vi "Apply TSC Pop Up.vi"(8 "error in":errorcluster, 9 "Material.Details in":T1={"Font Name"="Segoe UI", "Button.Font Size"=30, "Message.Font Size"=30, "Message.Justification"=enum."Center", "Picture Background"=16777216}, 10 "Theme":u16(ring)=3 items=["Light Theme", "Light Medium Contrast", "Light High Contrast", "Dark Theme", "Dark Medium Contrast", "Dark High Constrast"], 11 "Material Theme in":refnum<class "Material Theme.lvclass">) -> (0 "error out":errorcluster, 1 "Material.Details out":T1={"Font Name"="Segoe UI", "Button.Font Size"=30, "Message.Font Size"=30, "Message.Justification"=enum."Center", "Picture Background"=16777216}, 2 "Material.Scheme out":T2)   [LabVIEW 2021, in "TSC Material Theme.lvlib" / "Material Theme.lvclass"]
doc: "Apply a loaded theme to the TSC Pop Up Library.\n\nhttps://github.com/danielcoons/tsc-pop-up\n\n<b>Code Developed By:</b> +\nDaniel Coons +\nTechnology Service Corporation +\nwww.tsc.com/atcs"
uses:
  Material Theme.lvclass
  Material-Scheme/Material-Scheme.lvclass/Material-Scheme.ctl
  Material Theme.lvclass/Material Theme.ctl
  Material-Scheme/Material-Scheme.lvclass
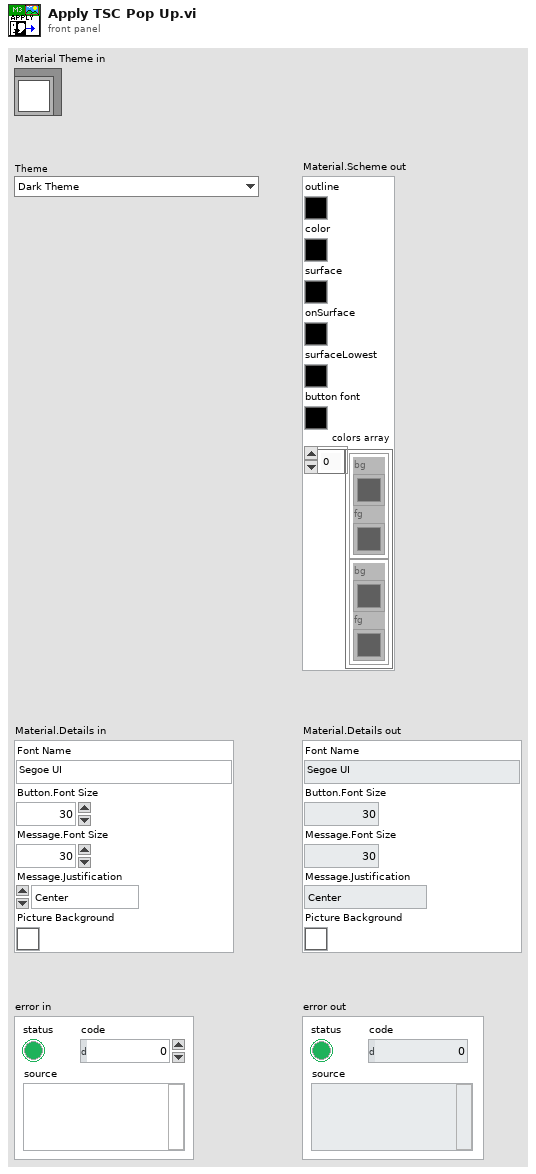
[diagram p1: front panel]
types:
  T1 = cluster{"Font Name":string, "Button.Font Size":u32, "Message.Font Size":u32, "Message.Justification":enum16{"Left", "Center", "Right"}, "Picture Background":u32}
  T2 = cluster{"outline":u32, "color":u32, "surface":u32, "onSurface":u32, "surfaceLowest":u32, "button font":u32, "colors array":cluster{"bg":u32, "fg":u32}[]}
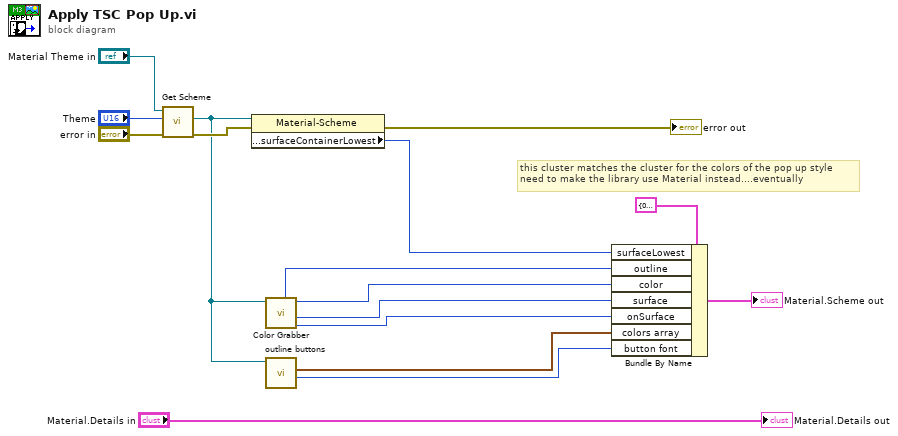
[diagram p0: block diagram]
diagram:
  # "this cluster matches the cluster for the colors of the pop up style\nneed to make the library use Material instead....eventually"
  n1 = call "Get Scheme.vi"("error in (no error)"="error in", "Theme"="Theme", "Material Theme in"="Material Theme in") -> ("error out"=w15:errorcluster, "Material-Scheme"=w10:refnum<class "Material-Scheme.lvclass">)  [unwired: 6 in, 1 out]
  n2 = property class="Material-Scheme"(reference=w10, error in=w15) -> (error out=→"error out":errorcluster, "data member access:Surface:surfaceContainerLowest"=w4:u32)  [unwired: 1 out]
  n3 = call "Color Grabber.vi"("Material-Scheme in"=w10) -> ("onSurface"=w5:u32, "surface"=w6:u32, "color"=w7:u32, "outline"=w8:u32)  [unwired: 4 in, 3 out]
  n4 = call "outline buttons.vi"("Material-Scheme in"=w10) -> ("font color"=w2:u32, "colors array"=w3:cluster{"bg":u32, "fg":u32}[])  [unwired: 9 in]
  n5 = Bundle By Name(cluster=T2 {"outline"=0, "color"=0, "surface"=0, "onSurface"=0, "surfaceLowest"=0, "button font"=0, "colors array"=[]} ("Material.Scheme out"), "surfaceLowest"=w4, "outline"=w8, "color"=w7, "surface"=w6, "onSurface"=w5, "colors array"=w3, "button font"=w2) -> (→"Material.Scheme out":T2)
  "Material.Details out" <- "Material.Details in"
